vi "moveZToInitialPos.vi"(8 "error in":errorcluster) -> (0 "error out":errorcluster)   [LabVIEW 2014]
doc: "André Romero - 2023\nandretec@ifsc.usp.br\nIFSC - USP"
uses:
  Global Motors.vi
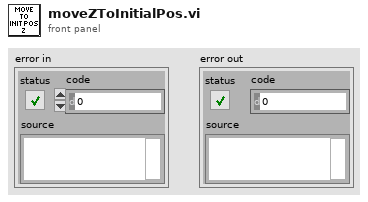
[diagram p1: front panel]
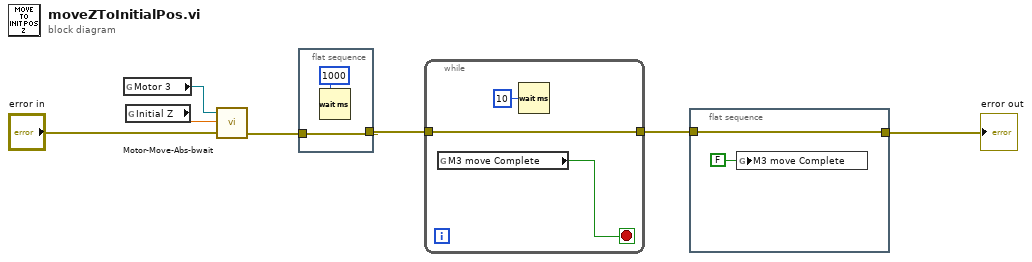
[diagram p0: block diagram]
diagram:
  n1 = global read "Global Motors.vi" "Motor 3"() -> (w3:refnum<k7>)
  n2 = global read "Global Motors.vi" "Initial Z"() -> (w4:dbl)
  n3 = call "Motor-Move-Abs-bwait.vi"("error"="error in", "Posição"=w4, "MG17Motor A"=w3) -> ("error out"=w6:errorcluster)  [unwired: 1 in, 1 out]
  n4 = flat-sequence {
    tunnel: w6 -> [w9]
    tunnel: [w9] -> w2
    frame #0 {
      n5 = Wait (ms)(milliseconds to wait=u32 1000) -> ()  [unwired: 1 out]
    }
  }
  n6 = while {
    tunnel: w2 -> [w12]
    tunnel: [w12] -> w5
    stop <- w10 stop-if-true
    n7 = global read "Global Motors.vi" "M3 move Complete"() -> (w10:bool)
    n8 = Wait (ms)(milliseconds to wait=u32 10) -> ()  [unwired: 1 out]
  }
  n9 = flat-sequence {
    tunnel: w5 -> [w13]
    tunnel: [w13] -> w7
    frame #0 {
      n10 = global write "Global Motors.vi" "M3 move Complete"(FALSE ("M1 move Complete")) -> ()
    }
  }
  "error out" <- w7
